vi "Log Event.vi"(8 "error in (no error)":errorcluster, 10 "Event Data":T1, 11 "Report Generator in":refnum<class "Report Generator.lvclass">) -> (0 "error out":errorcluster, 3 "Report Generator out":refnum<class "Report Generator.lvclass">)   [LabVIEW 2023, in "Report Generator.lvlib" / "Report Generator.lvclass"]
doc: "Descendant class must override this routine. \nAdd data record to Report\nEvent Data:\n<b>Time Stamp</b> The time at which the event occurred\n<b>Source</b> What device generated the event\n<b>Description</b> A description of the event\n<b>Details</b> Specific Details of the event."
uses:
  Library/Report Generator.lvclass
  Library/Report Generator.lvclass/Report Generator.ctl
  Custom Controls/Event Data.ctl
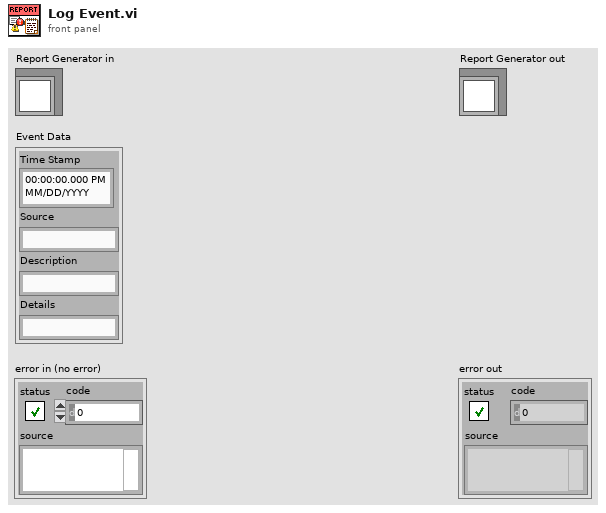
[diagram p1: front panel]
types:
  T1 = typedef "Report Generator.lvlib/Report Generator.lvclass/Event Data.ctl" = cluster{"Time Stamp":timestamp, "Source":string, "Description":string, "Details":string}
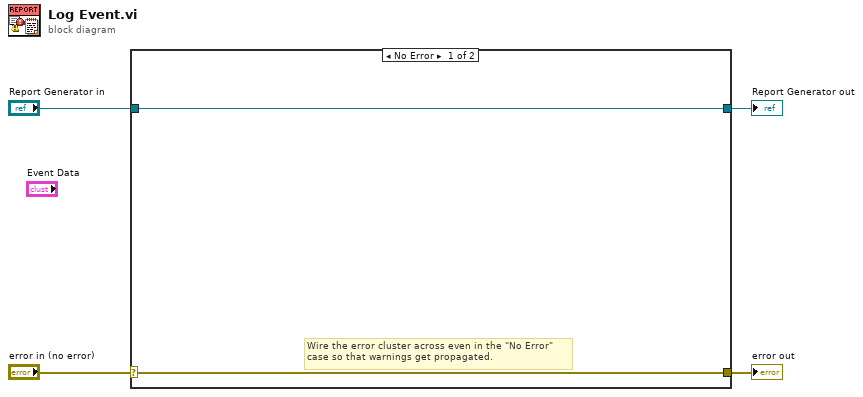
[diagram p0: block diagram]
diagram:
  n1 = case shown="No Error" "error in (no error)" {
    selector: "error in (no error)" -> [w5 w8]
    tunnel: [w5 w8] -> w3
    tunnel: [w6 w7] -> w1
    tunnel: "Report Generator in" -> [w6 w7]
    frame No Error {
      # "Wire the error cluster across even in the \"No Error\"\ncase so that warnings get propagated."
    }
    frame Error {
    }
  }
  "error out" <- w3
  "Report Generator out" <- w1
